vi "Simulator Cost Calculation.vi"(2 "Target Bonus":i16[](array[numeric]), 3 "Target Heading":i16, 4 "Candidate Valley Width":i16[](array[numeric]), 5 "Candidates":i16[](array[numeric]), 6 "Last Heading":i16, 7 "Current Heading":i16) -> (0 "Cost":dbl[](array[numeric]), 1 "Calculated Heading":i16)   [LabVIEW 2009]
panel:
  in  "F":dbl=50.0
  in  "Conv factor":i16
  in  "Calculated bearing vector":cluster{"x component":dbl, "y component":dbl}
  in  "E":dbl=50.0
  in  "D":dbl=1.0
  in  "C":dbl=1.0
  in  "B":dbl=2.0
  in  "A":dbl=3.0
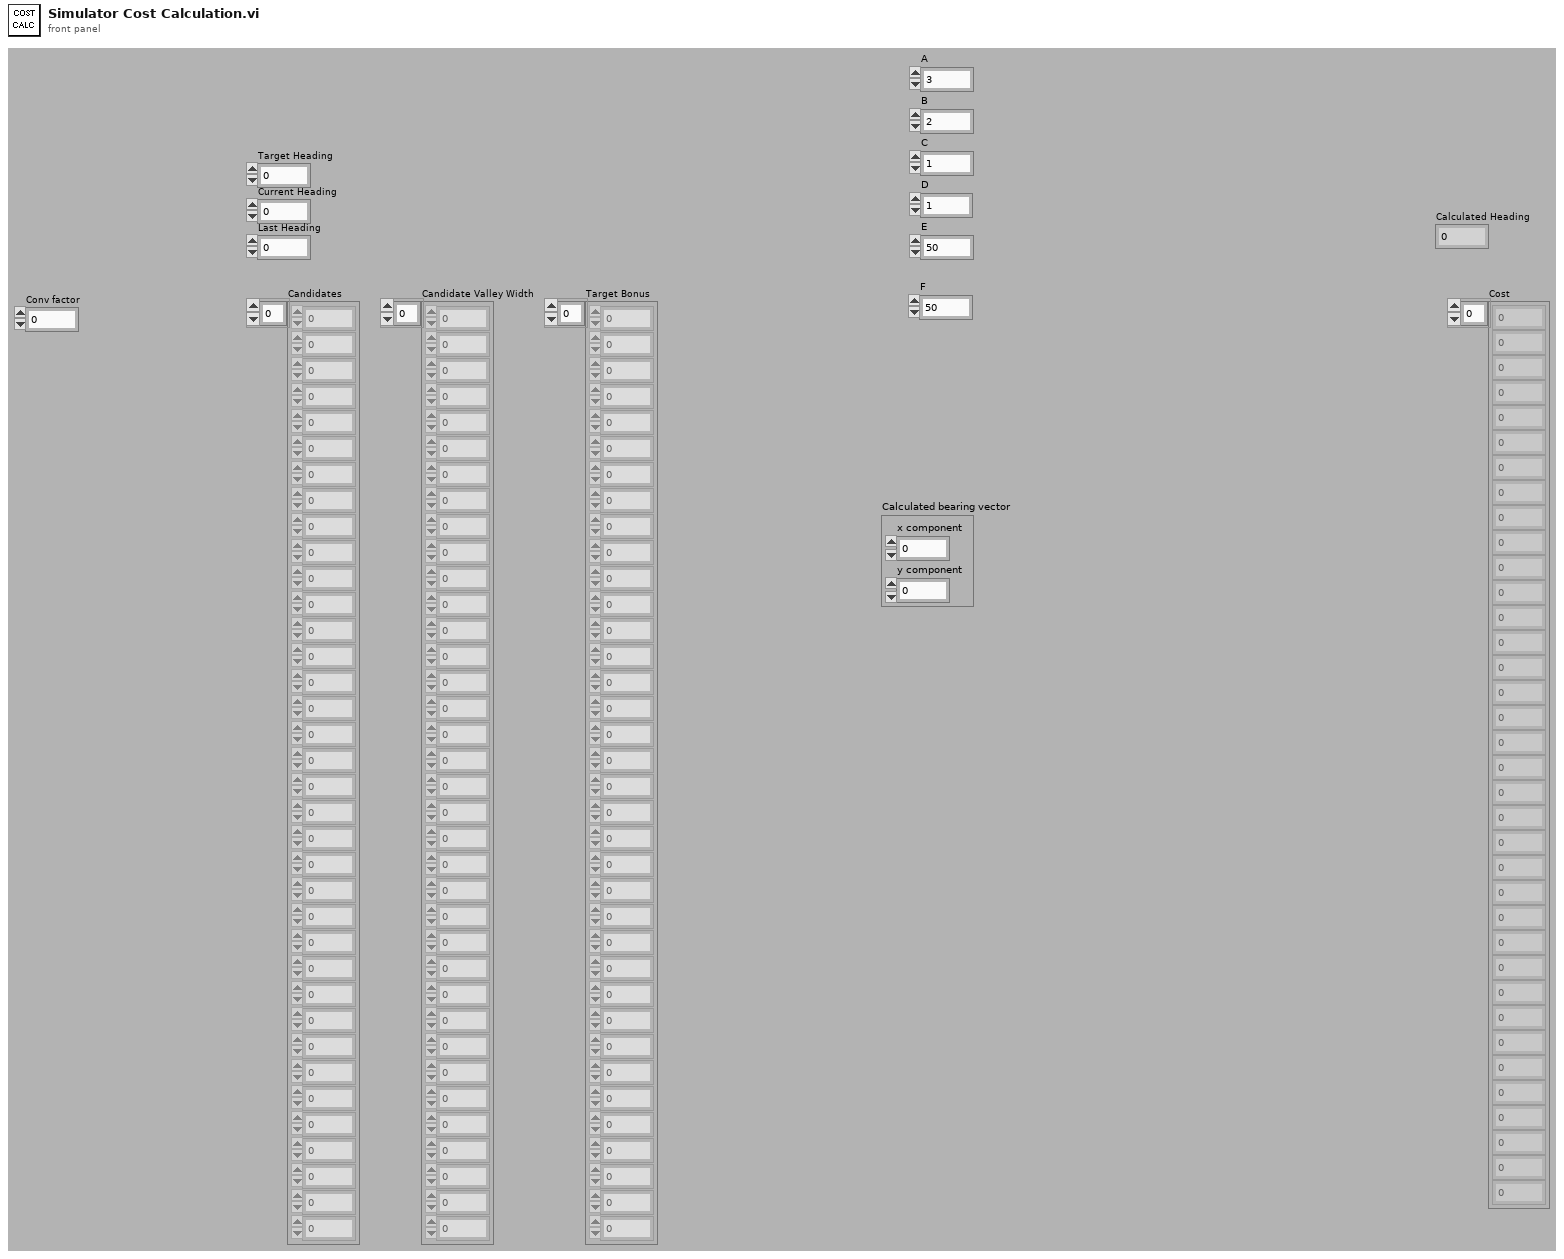
[diagram p1: front panel]
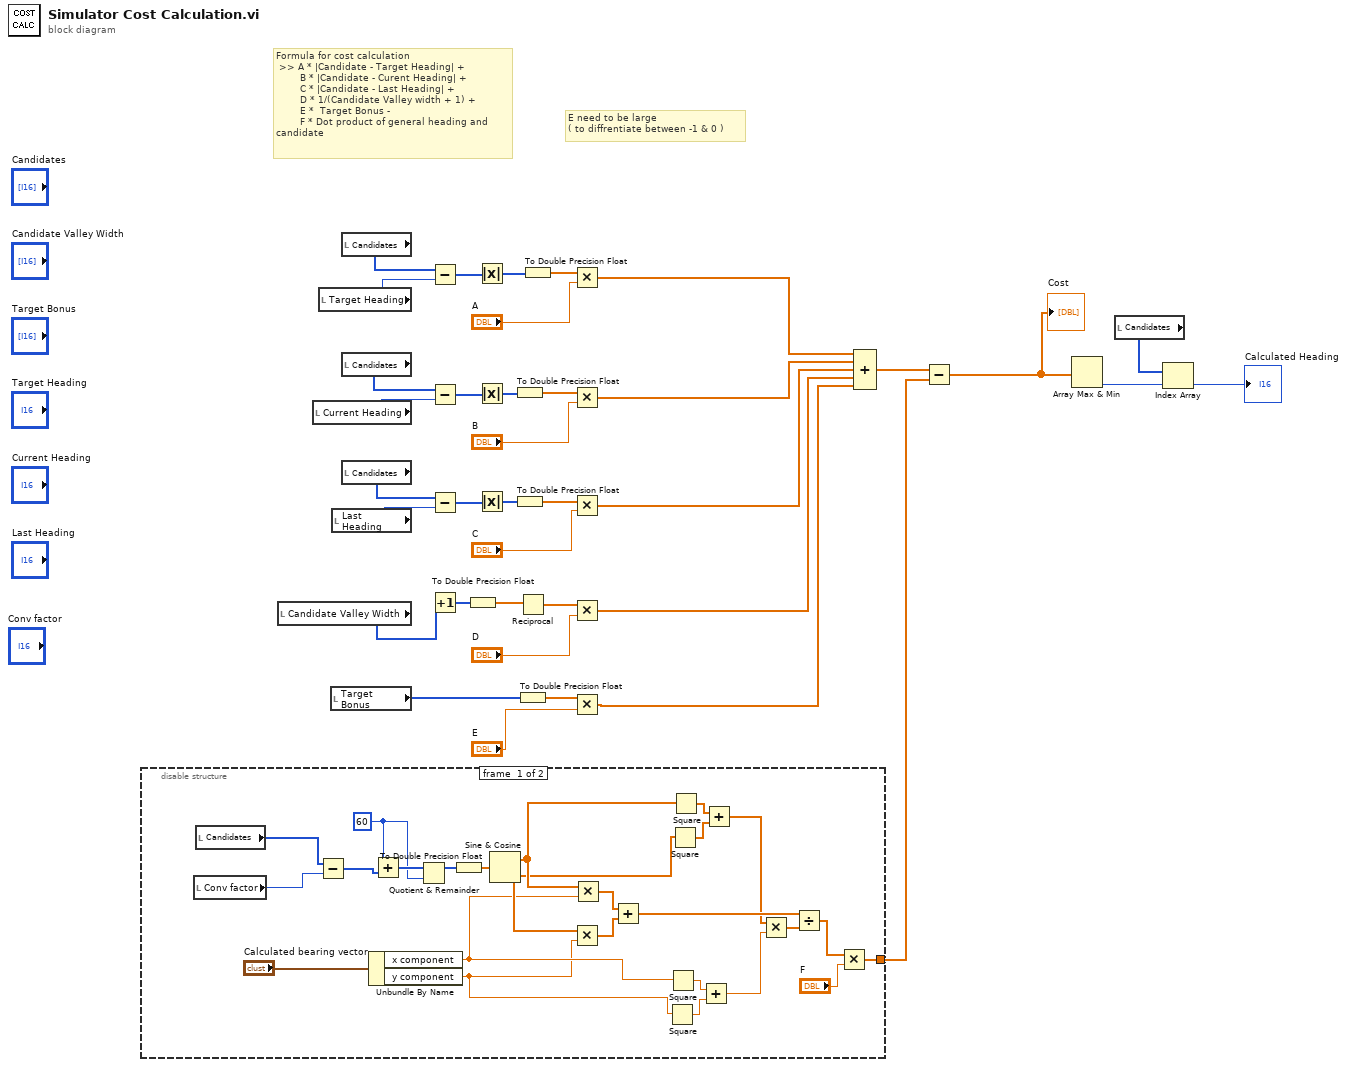
[diagram p0: block diagram]
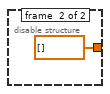
[diagram p2: hidden frame]
diagram:
  # "E need to be large\n( to diffrentiate between -1 & 0 )"
  # "Formula for cost calculation \n >> A * |Candidate - Target Heading| + \n        B * |Candidate - Curent Heading| + \n        C * |Candidate - Last Heading| +\n        D * 1/(Candidate Valley width + 1) +\n        E *  Target Bonus -\n        F * Dot product of general heading and candidate"
  n1 = disable-structure shown="Enabled" {
    disable-tunnel: [w38 dbl[] []] -> w1
    frame #0 {
      w61 = i16 60 ("y")
      n2 = local read "Conv factor"() -> (w59:i16)
      n3 = local read "Candidates"() -> (w58:i16[])
      n4 = Subtract(x=w58, y=w59) -> (x-y=w60:i16[])
      n5 = Unbundle By Name("Calculated bearing vector") -> ("x component"=w46:dbl, "y component"=w45:dbl)
      n6 = Add(x=w61, y=w60) -> (x+y=w62:i16[])
      n7 = Quotient & Remainder(x=w62, y=w61) -> (x-y*floor(x/y)=w57:i16[])  [unwired: 1 out]
      n8 = To Double Precision Float(number=w57) -> (double precision float=w56:dbl[])
      n9 = Sine & Cosine(0:w56) -> (1:w52:dbl[], 2:w51:dbl[])
      n10 = Multiply(x=w51, y=w45) -> (x*y=w53:dbl[])
      n11 = Multiply(x=w52, y=w46) -> (x*y=w54:dbl[])
      n12 = Add(x=w54, y=w53) -> (x+y=w44:dbl[])
      n13 = Square(x=w45) -> (x^2=w48:dbl)
      n14 = Square(x=w46) -> (x^2=w47:dbl)
      n15 = Square(x=w51) -> (x^2=w49:dbl[])
      n16 = Square(x=w52) -> (x^2=w50:dbl[])
      n17 = Add(x=w47, y=w48) -> (x+y=w42:dbl)
      n18 = Add(x=w50, y=w49) -> (x+y=w43:dbl[])
      n19 = Multiply(x=w43, y=w42) -> (x*y=w41:dbl[])
      n20 = Divide(x=w44, y=w41) -> (x/y=w39:dbl[])
      n21 = Multiply(x=w39, y="F") -> (x*y=w38:dbl[])
    }
    frame #1 {
    }
  }
  n22 = local read "Candidate Valley Width"() -> (w25:i16[])
  n23 = local read "Current Heading"() -> (w31:i16)
  n24 = local read "Target Heading"() -> (w36:i16)
  n25 = local read "Target Bonus"() -> (w10:i16[])
  n26 = local read "Last Heading"() -> (w27:i16)
  n27 = local read "Candidates"() -> (w37:i16[])
  n28 = local read "Candidates"() -> (w30:i16[])
  n29 = local read "Candidates"() -> (w26:i16[])
  n30 = Subtract(x=w37, y=w36) -> (x-y=w35:i16[])
  n31 = Subtract(x=w30, y=w31) -> (x-y=w32:i16[])
  n32 = Subtract(x=w26, y=w27) -> (x-y=w28:i16[])
  n33 = Increment(x=w25) -> (x+1=w13:i16[])
  n34 = To Double Precision Float(number=w13) -> (double precision float=w12:dbl[])
  n35 = Absolute Value(x=w35) -> (abs(x)=w18:i16[])
  n36 = Absolute Value(x=w32) -> (abs(x)=w17:i16[])
  n37 = Absolute Value(x=w28) -> (abs(x)=w14:i16[])
  n38 = To Double Precision Float(number=w17) -> (double precision float=w16:dbl[])
  n39 = To Double Precision Float(number=w14) -> (double precision float=w15:dbl[])
  n40 = Reciprocal(x=w12) -> (1/x=w23:dbl[])
  n41 = To Double Precision Float(number=w10) -> (double precision float=w11:dbl[])
  n42 = To Double Precision Float(number=w18) -> (double precision float=w19:dbl[])
  n43 = Multiply(x=w19, y="A") -> (x*y=w8:dbl[])
  n44 = Multiply(x=w16, y="B") -> (x*y=w7:dbl[])
  n45 = Multiply(x=w15, y="C") -> (x*y=w6:dbl[])
  n46 = Multiply(x=w23, y="D") -> (x*y=w5:dbl[])
  n47 = Multiply(x=w11, y="E") -> (x*y=w4:dbl[])
  n48 = Compound Arithmetic op=ADD(w8, w7, w6, w5, w4) -> (w2:dbl[])
  n49 = Subtract(x=w2, y=w1) -> (x-y=w3:dbl[])
  "Cost" <- w3
  n50 = Array Max & Min(array=w3) -> (min index (indices)=w20:i32)  [unwired: 3 out]
  n51 = local read "Candidates"() -> (w21:i16[])
  n52 = Index Array(array=w21, index=w20) -> (element=→"Calculated Heading":i16)
